vi "pdw 2 raw PDWs.vi"(8 "error in (no error)":errorcluster, 10 "PDWs":T1[](array[typedef]), 11 "device_type in":refnum<class "device_type.lvclass">) -> (0 "error out":errorcluster, 2 "Array":u64[][](array[numeric]), 3 "device_type out":refnum<class "device_type.lvclass">)   [LabVIEW 2021, in "device_type.lvclass"]
uses:
  device_type.lvclass
  pulse_tx_vis/PDW_lv2.ctl
  pulse_tx_vis/mode_type.ctl
  device_type.lvclass/device_type.ctl
  pulse_tx_vis/pdw.ctl
panel:
  out "lfm lost":bool
  out "mod too wide":bool
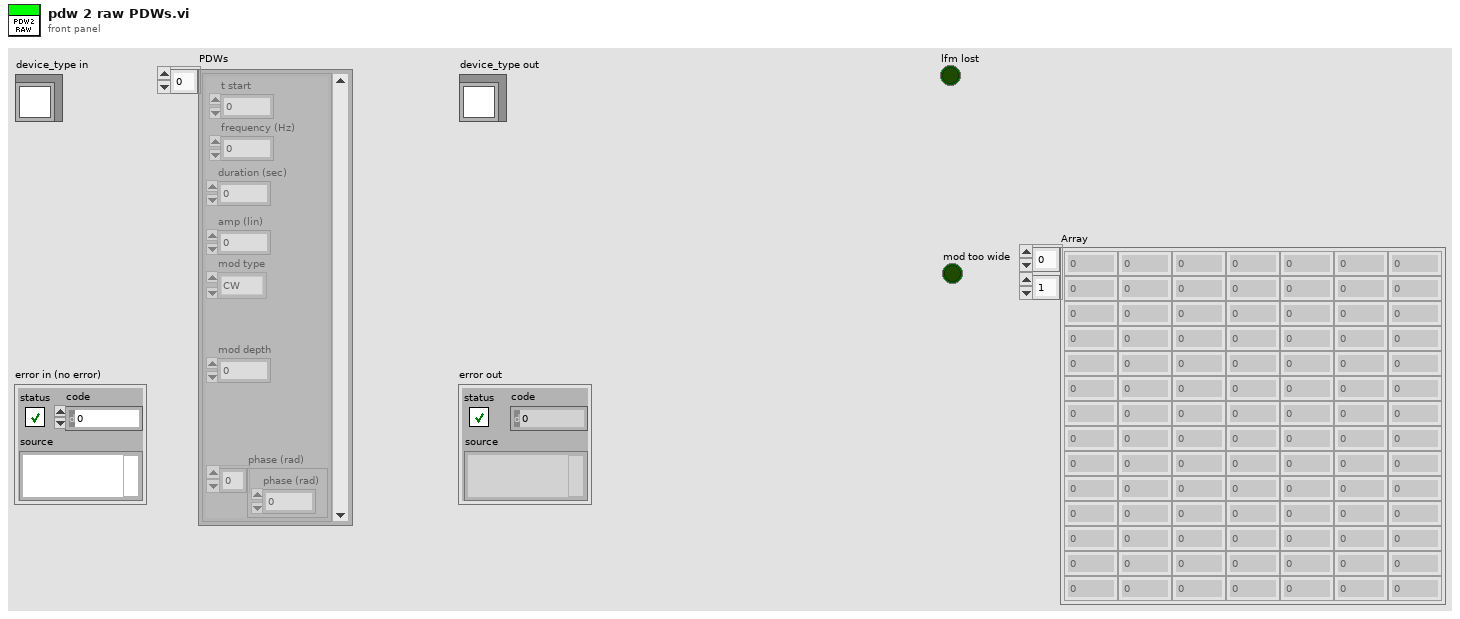
[diagram p1: front panel]
types:
  T1 = typedef "PDW_lv2.ctl" = cluster{"t start":dbl, "frequency (Hz)":dbl, "duration (sec)":dbl, "amp (lin)":dbl, "mod type":T2, "mod depth":dbl, "phase (rad)":dbl[]}
  T2 = typedef "mode_type.ctl" = enum8{"CW", "NC - CW", "NC - cw", "LFM", "BPSK", "QPSK"}
  T3 = typedef "pdw.ctl" = cluster{"PW":u32, "frequency shift":fxp<+/-,48,0>, "amp":fxp<+/-,18,1>, "mode type":T2, "mode depth":u32, "mode filter":u8, "phase shift":fxp<+/-,16,1>, "pulse shape filter":u8}
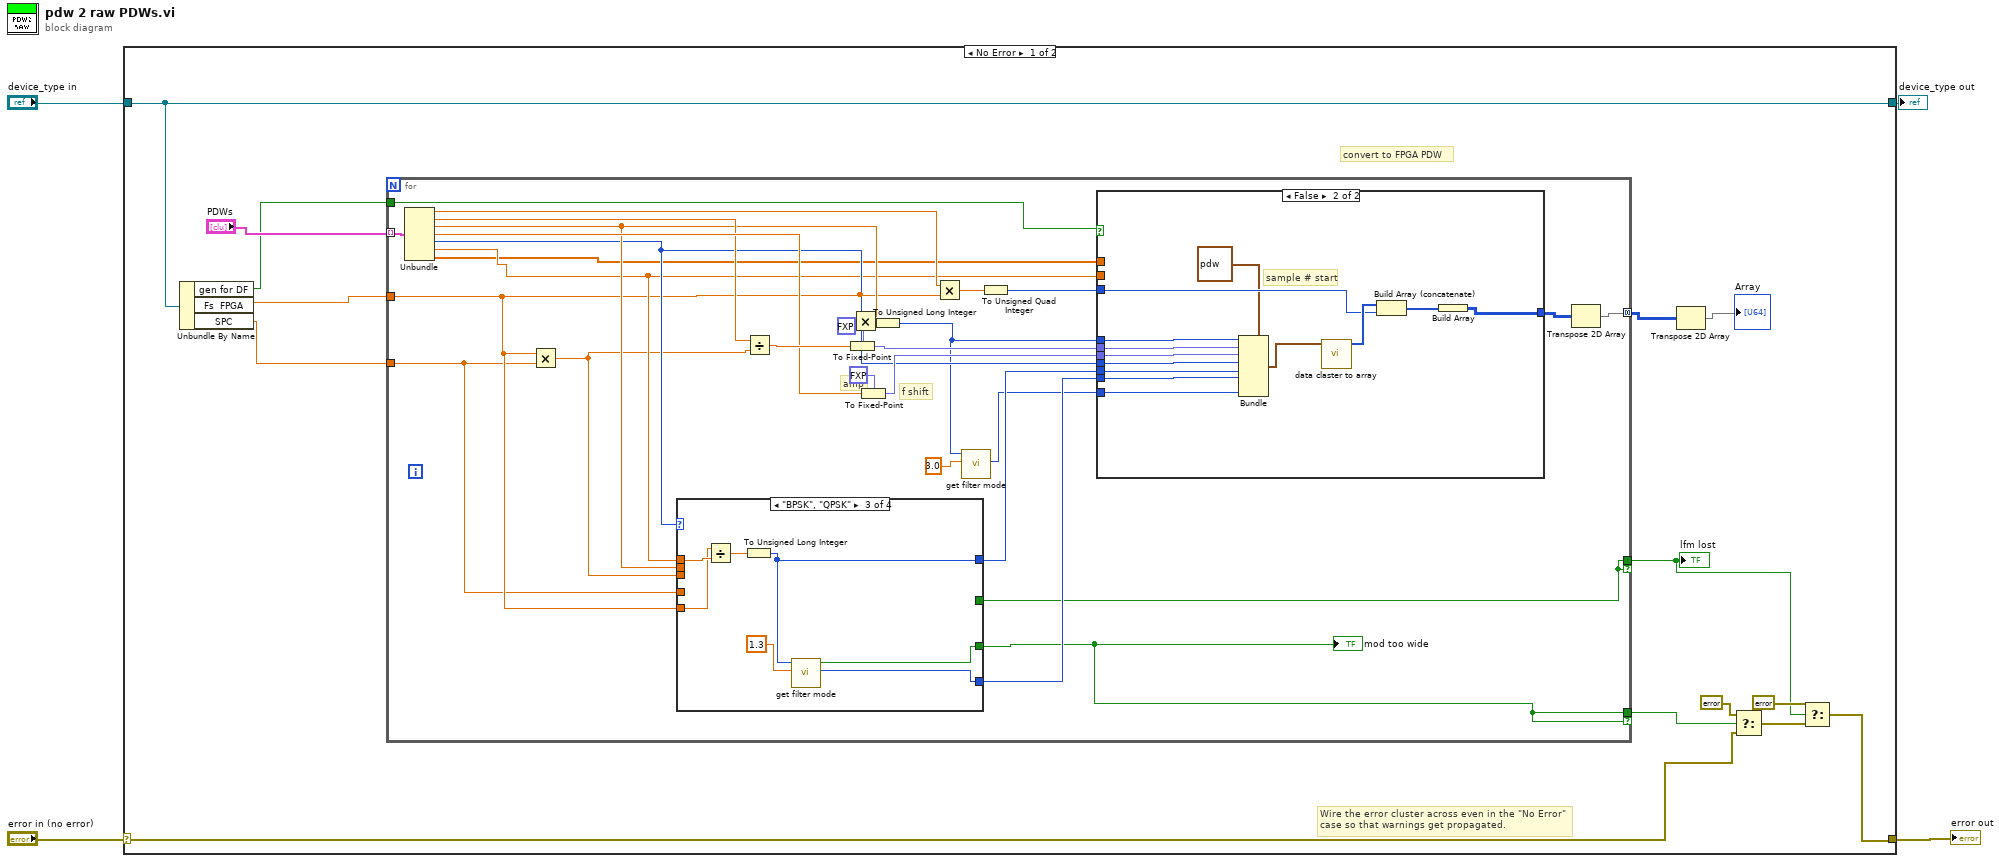
[diagram p0: block diagram]
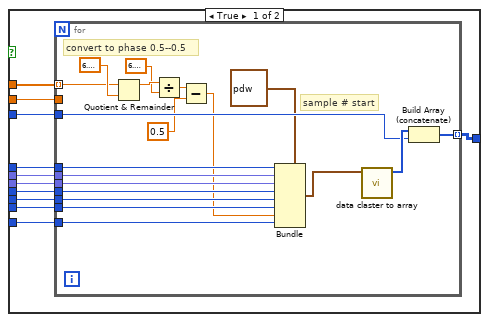
[diagram p2: hidden frame]
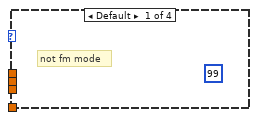
[diagram p3: hidden frame]
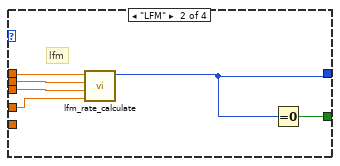
[diagram p4: hidden frame]
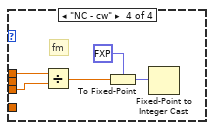
[diagram p5: hidden frame]
diagram:
  n1 = case shown="No Error" "error in (no error)" {
    selector: "error in (no error)" -> [w7 w110]
    tunnel: [w6 w110] -> w3
    tunnel: [w10 w109] -> w1
    tunnel: "device_type in" -> [w10 w109]
    frame No Error {
      # "convert to FPGA PDW"
      # "Wire the error cluster across even in the \"No Error\"\ncase so that warnings get propagated."
      n2 = Unbundle By Name(w10) -> ("gen for DF"=w5:bool, "Fs  FPGA"=w9:dbl, "SPC"=w8:dbl)
      n3 = for {
        tunnel: "PDWs" -> [w47] mode=indexing
        tunnel: [w29] -> w13 mode=concatenating
        tunnel: w9 -> [w24]
        tunnel: [w26] -> w11 if=w26
        tunnel: [w31] -> w16 if=w31
        tunnel: w8 -> [w23]
        tunnel: w5 -> [w19]
        # "amp"
        # "f shift"
        n4 = Unbundle(w47) -> ("t start"=w46:dbl, "frequency (Hz)"=w36:dbl, "duration (sec)"=w35:dbl, "amp (lin)"=w40:dbl, "mod type"=w34:T2, "mod depth"=w28:dbl, "phase (rad)"=w27:dbl[])
        n5 = Multiply(x=w24, y=w23) -> (x*y=w25:dbl)
        n6 = case shown="\"BPSK\", \"QPSK\"" w34 {
          tunnel: [_ w93 w100 _] -> w33
          tunnel: w25 -> [_ w96 _ w107]
          tunnel: w28 -> [_ w94 w103 w108]
          tunnel: w35 -> [_ w95 _ _]
          tunnel: [_ _ w101 _] -> w32
          tunnel: [_ _ w99 _] -> w31
          tunnel: [_ w92 _ _] -> w26
          tunnel: w24 -> [_ _ w98 _]
          tunnel: w23 -> [_ w91 _ _]
          frame Default {
            (unwired) u32 99 ("integer (fxp cast)")
            # "not fm mode"
          }
          frame "LFM" {
            # "lfm"
            n7 = call "lfm_rate_calculate.vi"("SPC"=w91, "fs"=w96, "pw"=w95, "f span"=w94) -> ("integer (fxp cast)"=w93:u32)  [unwired: 7 in]
            n8 = Equal To 0?(x=w93) -> (x = 0?=w92:bool)
          }
          frame "BPSK", "QPSK" {
            n9 = Divide(x=w98, y=w103) -> (x/y=w102:dbl)
            n10 = To Unsigned Long Integer(number=w102) -> (unsigned 32bit integer=w100:u32)
            n11 = call "get filter mode.vi"("filter rate"=1.3 ("y"), "Numeric in"=w100) -> ("filter mode"=w101:i32, "no fit filter"=w99:bool)  [unwired: 8 in]
          }
          frame "NC - cw" {
            # "fm"
            n12 = Divide(x=w108, y=w107) -> (x/y=w104:dbl)
            n13 = To Fixed-Point(fixed-point type=fxp<+,32,-16> 0.0, number=w104) -> (fixed-point=w106:fxp<+,32,-16>)
            n14 = Fixed-Point to Integer Cast(1:w106) -> ()  [unwired: 1 out]
          }
        }
        "mod too wide" <- w31
        n15 = Divide(x=w36, y=w25) -> (x/y=w44:dbl)
        n16 = To Fixed-Point(fixed-point type=fxp<+/-,48,0> 0.0 ("frequency shift"), number=w44) -> (fixed-point=w42:fxp<+/-,48,0>)
        n17 = Multiply(x=w35, y=w24) -> (x*y=w41:dbl)
        n18 = To Fixed-Point(fixed-point type=fxp<+/-,18,1> 0.0 ("I"), number=w40) -> (fixed-point=w38:fxp<+/-,18,1>)
        n19 = To Unsigned Long Integer(number=w41) -> (unsigned 32bit integer=w22:u32)
        n20 = Multiply(x=w46, y=w24) -> (x*y=w45:dbl)
        n21 = call "get filter mode.vi"("filter rate"=3.0, "Numeric in"=w22) -> ("filter mode"=w20:i32)  [unwired: 8 in, 1 out]
        n22 = To Unsigned Quad Integer(1:w45) -> (0:w37:u64)
        n23 = case shown="False" w19 {
          tunnel: w42 -> [w58 w90]
          tunnel: w38 -> [w57 w89]
          tunnel: w37 -> [w56 w87]
          tunnel: [w55 w80] -> w30
          tunnel: w22 -> [w54 w84]
          tunnel: w34 -> [w53 w83]
          tunnel: w33 -> [w52 w79]
          tunnel: w32 -> [w51 w82]
          tunnel: w28 -> [w50 _]
          tunnel: w27 -> [w49 _]
          tunnel: w20 -> [w48 w78]
          frame True {
            n24 = for {
              tunnel: w58 -> [w77]
              tunnel: w57 -> [w76]
              tunnel: w56 -> [w74]
              tunnel: [w71] -> w55 mode=indexing
              tunnel: w54 -> [w70]
              tunnel: w53 -> [w69]
              tunnel: w52 -> [w68]
              tunnel: w51 -> [w67]
              tunnel: w50 -> [_]
              tunnel: w49 -> [w60] mode=indexing
              tunnel: w48 -> [w59]
              # "convert to phase 0.5--0.5"
              # "sample # start"
              n25 = Quotient & Remainder(x=w60, y=6.283185307179586) -> (x-y*floor(x/y)=w65:dbl)  [unwired: 1 out]
              n26 = Divide(x=w65, y=6.283185307179586) -> (x/y=w63:dbl)
              n27 = Subtract(x=w63, y=0.5) -> (x-y=w61:dbl)
              n28 = Bundle(cluster=T3 {"PW"=0, "frequency shift"=0.0, "amp"=0.0, "mode type"=enum."CW", "mode depth"=0, "mode filter"=0, "phase shift"=0.0, "pulse shape filter"=0} ("Cluster"), "PW"=w70, "frequency shift"=w77, "amp"=w76, "mode type"=w69, "mode depth"=w68, "mode filter"=w67, "phase shift"=w61, "pulse shape filter"=w59) -> (w72:T3)
              n29 = call "data claster to array.vi"("Cluster"=w72) -> ("Array"=w75:u64[])  [unwired: 10 in]
              n30 = Build Array (concatenate)(w75, w74) -> (w71:u64[])
            }
          }
          frame False {
            # "sample # start"
            n31 = Bundle(cluster=T3 {"PW"=0, "frequency shift"=0.0, "amp"=0.0, "mode type"=enum."CW", "mode depth"=0, "mode filter"=0, "phase shift"=0.0, "pulse shape filter"=0} ("Cluster"), "PW"=w84, "frequency shift"=w90, "amp"=w89, "mode type"=w83, "mode depth"=w79, "mode filter"=w82, "pulse shape filter"=w78) -> (w85:T3)  [unwired: 1 in]
            n32 = call "data claster to array.vi"("Cluster"=w85) -> ("Array"=w88:u64[])  [unwired: 10 in]
            n33 = Build Array (concatenate)(w88, w87) -> (w81:u64[])
            n34 = Build Array(w81) -> (w80:u64[][])
          }
        }
        n35 = Transpose 2D Array(2D array=w30) -> (transposed array=w29:u64[][])
      }
      "lfm lost" <- w11
      n36 = Transpose 2D Array(2D array=w13) -> (transposed array=→"Array":u64[][])
      n37 = Select(t=errorcluster {"status"=TRUE, "code"=5432, "source"="PSK mod too wide"} ("error out"), s=w16, f=w7) -> (s? t:f=w15:errorcluster)
      n38 = Select(t=errorcluster {"status"=TRUE, "code"=5432, "source"="The LFM value lost, pls take higher value for it"} ("error out"), s=w11, f=w15) -> (s? t:f=w6:errorcluster)
    }
    frame Error {
    }
  }
  "error out" <- w3
  "device_type out" <- w1
